vi "test io.vi"(1 "Call Context":T8) -> (0 "Test Data":T9)   [LabVIEW 2013]
uses:
  typedefs/test/test data.ctl
  <vilib>/Rock Robotics/WPI/DriverStation/WPI_DriverStationDerivedRobotMode.ctl
  <vilib>/Rock Robotics/WPI/Compressor/WPI_CompressorDevRef.ctl
  <vilib>/Rock Robotics/WPI/DigitalInput/WPI_DigitalInputDevRef.ctl
  <vilib>/Rock Robotics/SystemInterfaces/DIO/FPGA_DIOChannel.ctl
  <vilib>/Rock Robotics/SystemInterfaces/Typedef/FPGA_TypedefDigitalModule.ctl
  <vilib>/Rock Robotics/WPI/Relay/WPI_RelayDevRef.ctl
  <vilib>/Rock Robotics/SystemInterfaces/DIO/FPGA_DIORelayChannel.ctl
  <vilib>/Rock Robotics/WPI/Relay/WPI_RelayDirection.ctl
  typedefs/fg_getset.ctl
  <vilib>/Rock Robotics/WPI/Solenoid/WPI_SolenoidGetEnum.vi
  <vilib>/Rock Robotics/WPI/Compressor/WPI_CompressorGetSetRefNum.vi
panel:
  out "resetDrive":bool
  out "Compressor":bool
  out "CompressorDevRef":T1={"DevStatus"={"status"=FALSE, "code"=0, "source"=""}, "DigitalInputDevRef"={"DevStatus"={"status"=FALSE, "code"=0, "source"=""}, "DIO Channel"=enum."DIO 1", "Digital Module"=enum."Digital Module 1"}, "RelayDevRef"={"DevStatus"={"status"=FALSE, "code"=0, "source"=""}, "Relay Channel"=enum."Invalid", "Digital Module"=enum."Digital Module 1", "Relay Direction"=enum."Both directions"}}
  # "Get Test Data"
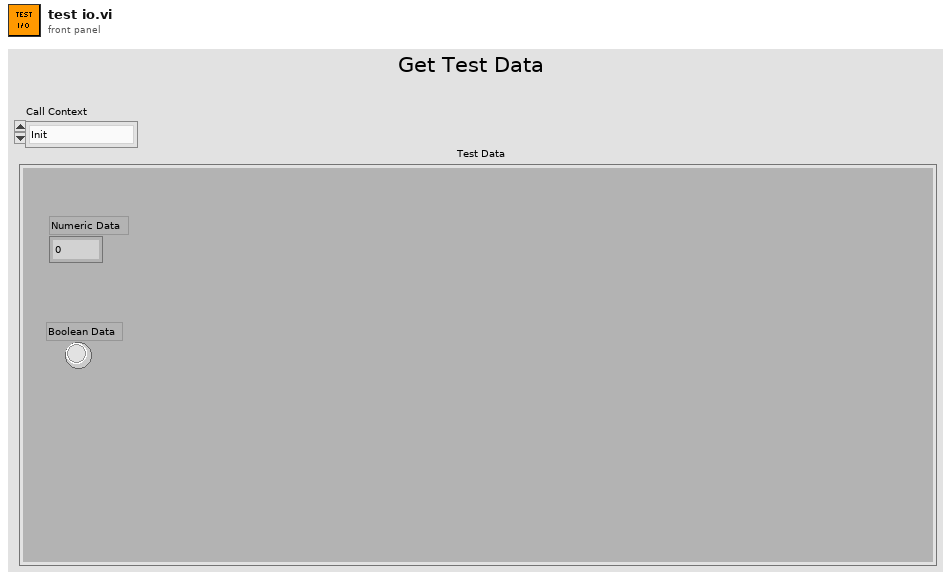
[diagram p1: front panel]
types:
  T1 = typedef "WPI_CompressorDevRef.ctl" = cluster{"DevStatus":errorcluster, "DigitalInputDevRef":T2, "RelayDevRef":T5}
  T2 = typedef "WPI_DigitalInputDevRef.ctl" = cluster{"DevStatus":errorcluster, "DIO Channel":T3, "Digital Module":T4}
  T3 = typedef "FPGA_DIOChannel.ctl" = enum8{"DIO 1", "DIO 2", "DIO 3", "DIO 4", "DIO 5", "DIO 6", "DIO 7", "DIO 8", "DIO 9", "DIO 10", "DIO 11", "DIO 12", "DIO 13", "DIO 14", "Invalid"}
  T4 = typedef "FPGA_TypedefDigitalModule.ctl" = enum16{"Digital Module 1", "Digital Module 2"}
  T5 = typedef "WPI_RelayDevRef.ctl" = cluster{"DevStatus":errorcluster, "Relay Channel":T6, "Digital Module":T4, "Relay Direction":T7}
  T6 = typedef "FPGA_DIORelayChannel.ctl" = enum8{"Relay 1", "Relay 2", "Relay 3", "Relay 4", "Relay 5", "Relay 6", "Relay 7", "Relay 8", "Invalid"}
  T7 = typedef "WPI_RelayDirection.ctl" = enum16{"Both directions", "Forward only", "Reverse only"}
  T8 = typedef "WPI_DriverStationDerivedRobotMode.ctl" = enum16{"Init", "Execute", "Stop"}
  T9 = typedef "test data.ctl" = cluster{"Numeric Data":dbl, "Boolean Data":bool}
  T10 = typedef "fg_getset.ctl" = enum16{"Get", "Set"}
  T11 = typedef "WPI_SolenoidDevRef.ctl" = cluster{"DevStatus":errorcluster, "Solenoid Module":T12, "Forward Solenoid Channel":T13, "Reverse Solenoid Channel":T13}
  T12 = typedef "FPGA_TypedefSolenoidModule.ctl" = enum16{"Solenoid Module 1", "Solenoid Module 2"}
  T13 = typedef "WPI_SolenoidChannel.ctl" = enum8{"Solenoid 1", "Solenoid 2", "Solenoid 3", "Solenoid 4", "Solenoid 5", "Solenoid 6", "Solenoid 7", "Solenoid 8", "Invalid"}
  T14 = typedef "WPI_EncoderDevRef.ctl" = cluster{"DevStatus":errorcluster, "EncoderIndex":T15, "CounterIndex":T16, "DistancePerCount":dbl, "Decoding Type":T17}
  T15 = typedef "FPGA_EncoderIdx.ctl" = enum8{"Enc 0", "Enc 1", "Enc 2", "Enc 3", "Invalid"}
  T16 = typedef "FPGA_CounterCtrSystemIndex.ctl" = enum8{"Ctr 0", "Ctr 1", "Ctr 2", "Ctr 3", "Ctr 4", "Ctr 5", "Ctr 6", "Ctr 7", "Invalid"}
  T17 = typedef "WPI_EncoderType.ctl" = enum16{"1x", "2x", "4x"}
  T18 = typedef "test controls.ctl" = cluster{"Button":bool, "Switch":bool, "Slider":dbl}
  T19 = typedef "WPI_SolenoidValue.ctl" = enum16{"Off", "On", "Forward", "Reverse"}
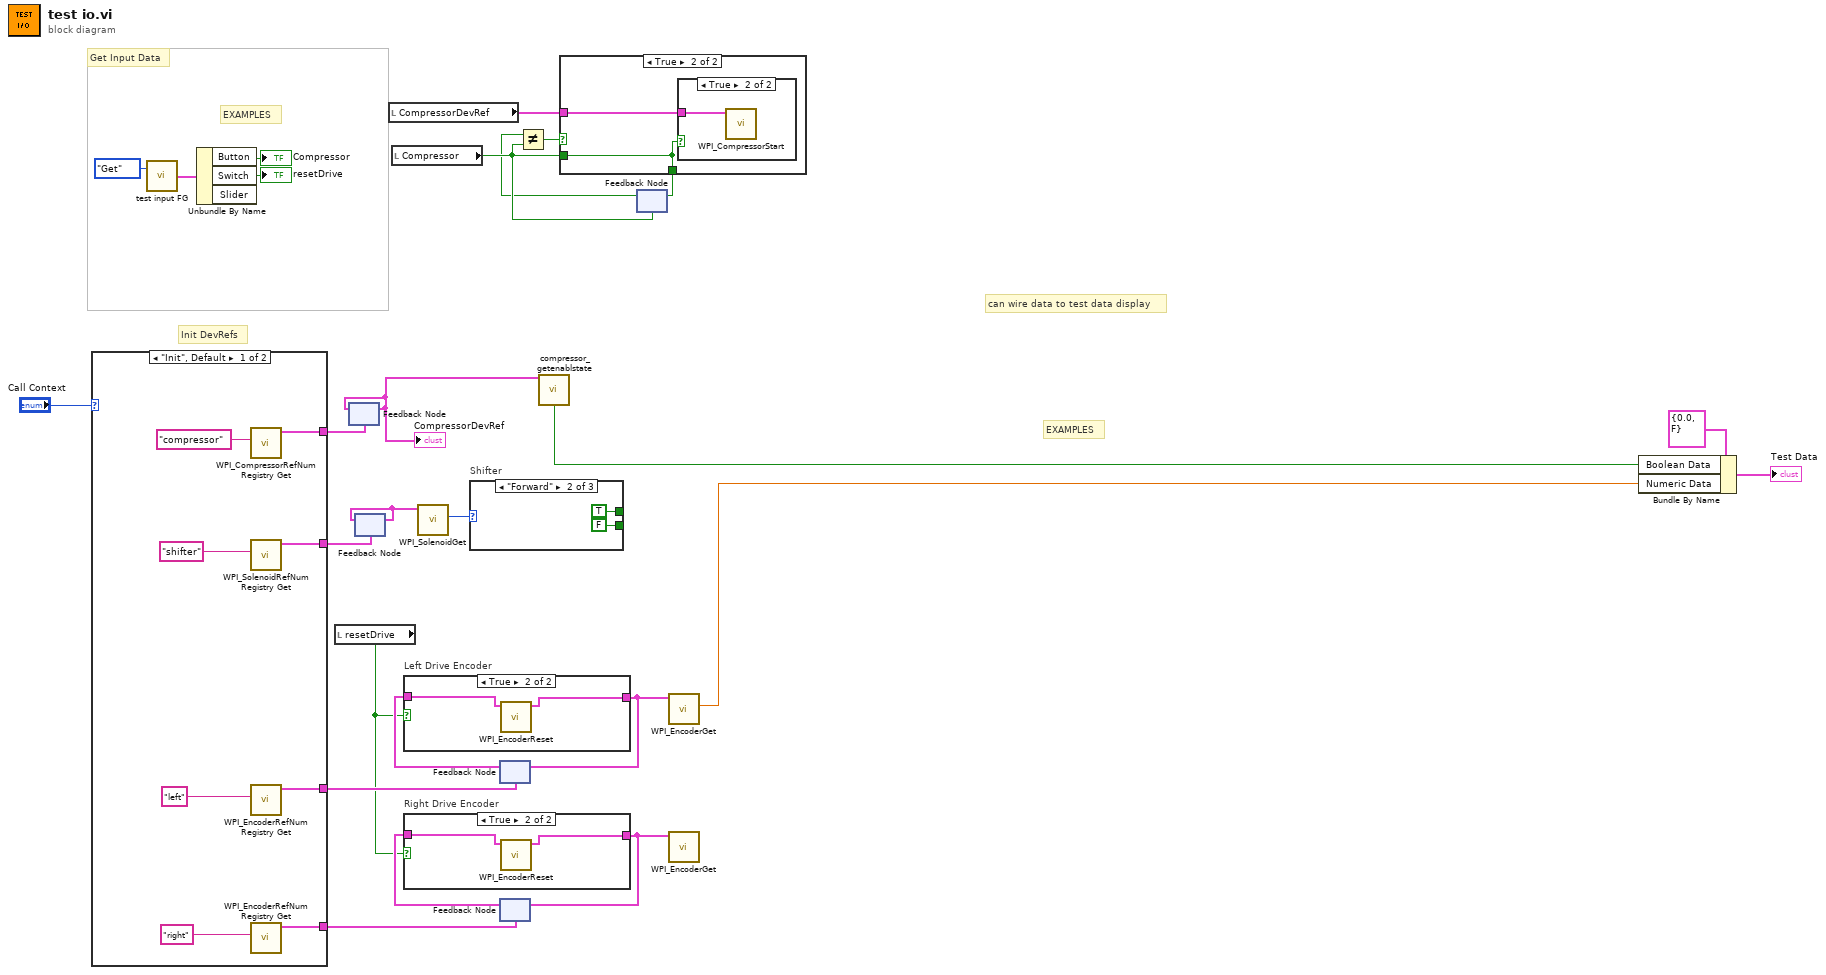
[diagram p0: block diagram]
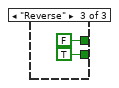
[diagram p5: hidden frame]
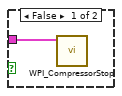
[diagram p7: hidden frame]
diagram:
  # "EXAMPLES"
  # "can wire data to test data display"
  # "EXAMPLES"
  # "Init DevRefs"
  # "Get Input Data"
  n1 = case shown="\"Init\", Default" "Call Context" {
    tunnel: [w34 _] -> w24
    tunnel: [w31 _] -> w12
    tunnel: [w30 _] -> w6
    tunnel: [w29 _] -> w5
    frame "Init", Default {
      n2 = call <vilib>:"WPI_CompressorRefNum Registry Get.vi"("refnum name"="compressor") -> ("CompressorDevRef"=w34:T1)  [unwired: 9 in, 1 out]
      n3 = call <vilib>:"WPI_SolenoidRefNum Registry Get.vi"("refnum name"="shifter") -> ("SolenoidDevRef"=w31:T11)  [unwired: 9 in, 1 out]
      n4 = call <vilib>:"WPI_EncoderRefNum Registry Get.vi"("refnum name"="left") -> ("EncoderDevRef"=w30:T14)  [unwired: 9 in, 1 out]
      n5 = call <vilib>:"WPI_EncoderRefNum Registry Get.vi"("refnum name"="right") -> ("EncoderDevRef"=w29:T14)  [unwired: 9 in, 1 out]
    }
    frame "Execute", "Stop" {
      # "do nothing"
    }
  }
  n6 = call "test input FG.vi"("Menu"=fg_getset."Get") -> ("Test Controls Out"=w16:T18)  [unwired: 1 in]
  n7 = Unbundle By Name(w16) -> ("Button"=→"Compressor":bool, "Switch"=→"resetDrive":bool)  [unwired: 1 out]
  n8 = local read "resetDrive"() -> (w3:bool)
  n9 = feedback #1(w24) -> (w11:T1)
  "CompressorDevRef" <- w11
  n10 = feedback-in #1(w11) -> ()
  n11 = feedback #2(w12) -> (w13:T11)
  n12 = feedback-in #2(w13) -> ()
  n13 = local read "CompressorDevRef"() -> (w22:T1)
  n14 = local read "Compressor"() -> (w21:bool)
  n15 = call-poly <vilib>:"WPI_SolenoidGet.vi"("SolenoidDevRef"=w13) -> ("Value"=w14:T19)  [unwired: 8 in, 2 out]
  n16 = case "Shifter" shown="\"Forward\"" w14 {
    tunnel: [_ TRUE FALSE] -> _
    tunnel: [_ FALSE TRUE] -> _
    frame "Off", Default {
    }
    frame "Forward" {
    }
    frame "Reverse" {
    }
  }
  n17 = feedback #3(w6) -> (w7:T14)
  n18 = case "Left Drive Encoder" shown="True" w3 {
    tunnel: w7 -> [w39 w41]
    tunnel: [w39 w40] -> w9
    frame False {
    }
    frame True {
      n19 = call <vilib>:"WPI_EncoderReset.vi"("EncoderDevRef"=w41) -> ("EncoderDevRef"=w40:T14)  [unwired: 9 in, 1 out]
    }
  }
  n20 = feedback-in #3(w9) -> ()
  n21 = feedback #4(w5) -> (w8:T14)
  n22 = case "Right Drive Encoder" shown="True" w3 {
    tunnel: w8 -> [w42 w44]
    tunnel: [w42 w43] -> w10
    frame False {
    }
    frame True {
      n23 = call <vilib>:"WPI_EncoderReset.vi"("EncoderDevRef"=w44) -> ("EncoderDevRef"=w43:T14)  [unwired: 9 in, 1 out]
    }
  }
  n24 = feedback-in #4(w10) -> ()
  n25 = call "compressor_getenablstate.vi"("CompressorDevRef"=w11) -> ("Charging"=w2:bool)  [unwired: 8 in, 6 out]
  n26 = feedback #5(w21) -> (w20:bool)
  n27 = Not Equal?(x=w20, y=w21) -> (x != y?=w19:bool)
  n28 = case shown="True" w19 {
    tunnel: w21 -> [w45 w47]
    tunnel: [w45 w47] -> w18
    tunnel: w22 -> [_ w46]
    frame False {
    }
    frame True {
      n29 = case shown="True" w47 {
        tunnel: w46 -> [w48 w49]
        frame False {
          n30 = call <vilib>:"WPI_CompressorStop.vi"("CompressorDevRef"=w48) -> ()  [unwired: 9 in, 2 out]
        }
        frame True {
          n31 = call <vilib>:"WPI_CompressorStart.vi"("CompressorDevRef"=w49) -> ()  [unwired: 9 in, 2 out]
        }
      }
    }
  }
  n32 = feedback-in #5(w18) -> ()
  n33 = call <vilib>:"WPI_EncoderGet.vi"("EncoderDevRef"=w9) -> ("Distance"=w1:dbl)  [unwired: 5 in, 5 out]
  n34 = call <vilib>:"WPI_EncoderGet.vi"("EncoderDevRef"=w10) -> ()  [unwired: 5 in, 6 out]
  n35 = Bundle By Name(cluster=T9 {"Numeric Data"=0.0, "Boolean Data"=FALSE} ("Test Data"), "Boolean Data"=w2, "Numeric Data"=w1) -> (→"Test Data":T9)
